vi "TPP-printer-v3.2.vi"() -> ()   [LabVIEW 2015]
uses:
  <vilib>/Math Plots/3D Math Plots/3D Scatter/3D Scatter XCtrl/3D Scatter.xctl
  <vilib>/DAQmx/write.llb/DAQmx Write (Digital Bool 1Line 1Point).vi
  <vilib>/Utility/file.llb/Read Delimited Spreadsheet (I64).vi
  <vilib>/Math Plots/3D Math Plots/3D Scatter/3D Scatter Datatype/Public/Plot Helper (Vector).vi
  <vilib>/DAQmx/create/channels.llb/DAQmx Create Channel (DO-Digital Output).vi
  <vilib>/DAQmx/miscellaneous.llb/DAQmx Fill In Error Info.vi
  <vilib>/Math Plots/3D Math Plots/3D Scatter/3D Scatter Datatype/3D Scatter Datatype.lvclass
panel:
  in  "Z轴驱动序列号":string="27002049"
  out "当前状态：":string
  in  "停止":bool
  in  "选项卡控件":enum32{"参数设置", "模型预览", "打印监控", "信息反馈"}(tab)
  in  "打印设置":T1={"f_objecitve(mm)"=1.8, "f_tubelens(mm)"=200.0, "f_scanlens(mm)"=50.0, "模型高/um"=2.0, "XY速度(um/s) "=0.0, "比例因子(V/°)"=1.0}
  in  "I/O 设置":T2={"matlab函数目录"=path "C:/Users/eason/Documents/GitHub/TPP-3D-printer/Matlab", "读取点阵文件"=path "C:/Users/eason/Documents/GitHub/TPP-3D-printer/Matlab/grating.txt", "DO通道：shutter控制"="Dev1/port1/line0", "AO通道：X前Y后"="Dev1/ao0:1", "Z轴驱动序列号"="27002049"}
  in  "刷新设置":bool
  out "三维散点图":refnum<class "3D Plot Datatype.lvclass">[](xcontrol)
  in  "取消打印":bool
  in  "开始打印":bool
  out "XYZG当前值/um":dbl[](array[numeric])=[-6.2105263157894735, -0.5263157894736842, 0.0, 1.0] format="%#.2g"
  out "每点耗时/ms":dbl=12.012958526611328 format="%#.0f"
  out "每行耗时/s":dbl=1.5567584037780762 format="%#.2g"
  out "每层耗时/min":dbl format="%#.2g"
  out "当前完成量：":u8(slide)=3 scale=0.0..100.0
  out "%":dbl=3.284878476249388 format="%#.2g"
  out "耗时/min":dbl=1.0008915185928344 format="%#.2g"
  out "三维散点图 2":refnum<class "3D Plot Datatype.lvclass">[](xcontrol)
  in  "跟踪路径":bool
  out "时刻":T3={"点时间"=timestamp(3595558893.17812 s since 1904-01-01), "行时间"=timestamp(3595558891.757594 s since 1904-01-01), "层时间"=timestamp(3595558833.124629 s since 1904-01-01)}
  out "起始时间":timestamp
  out "暂停时间/min":dbl=1.0008915185928344 format="%#.2g"
  out "当前扫描速度(um/s)":dbl
  out "XYZG坐标表":dbl[][](array[numeric])
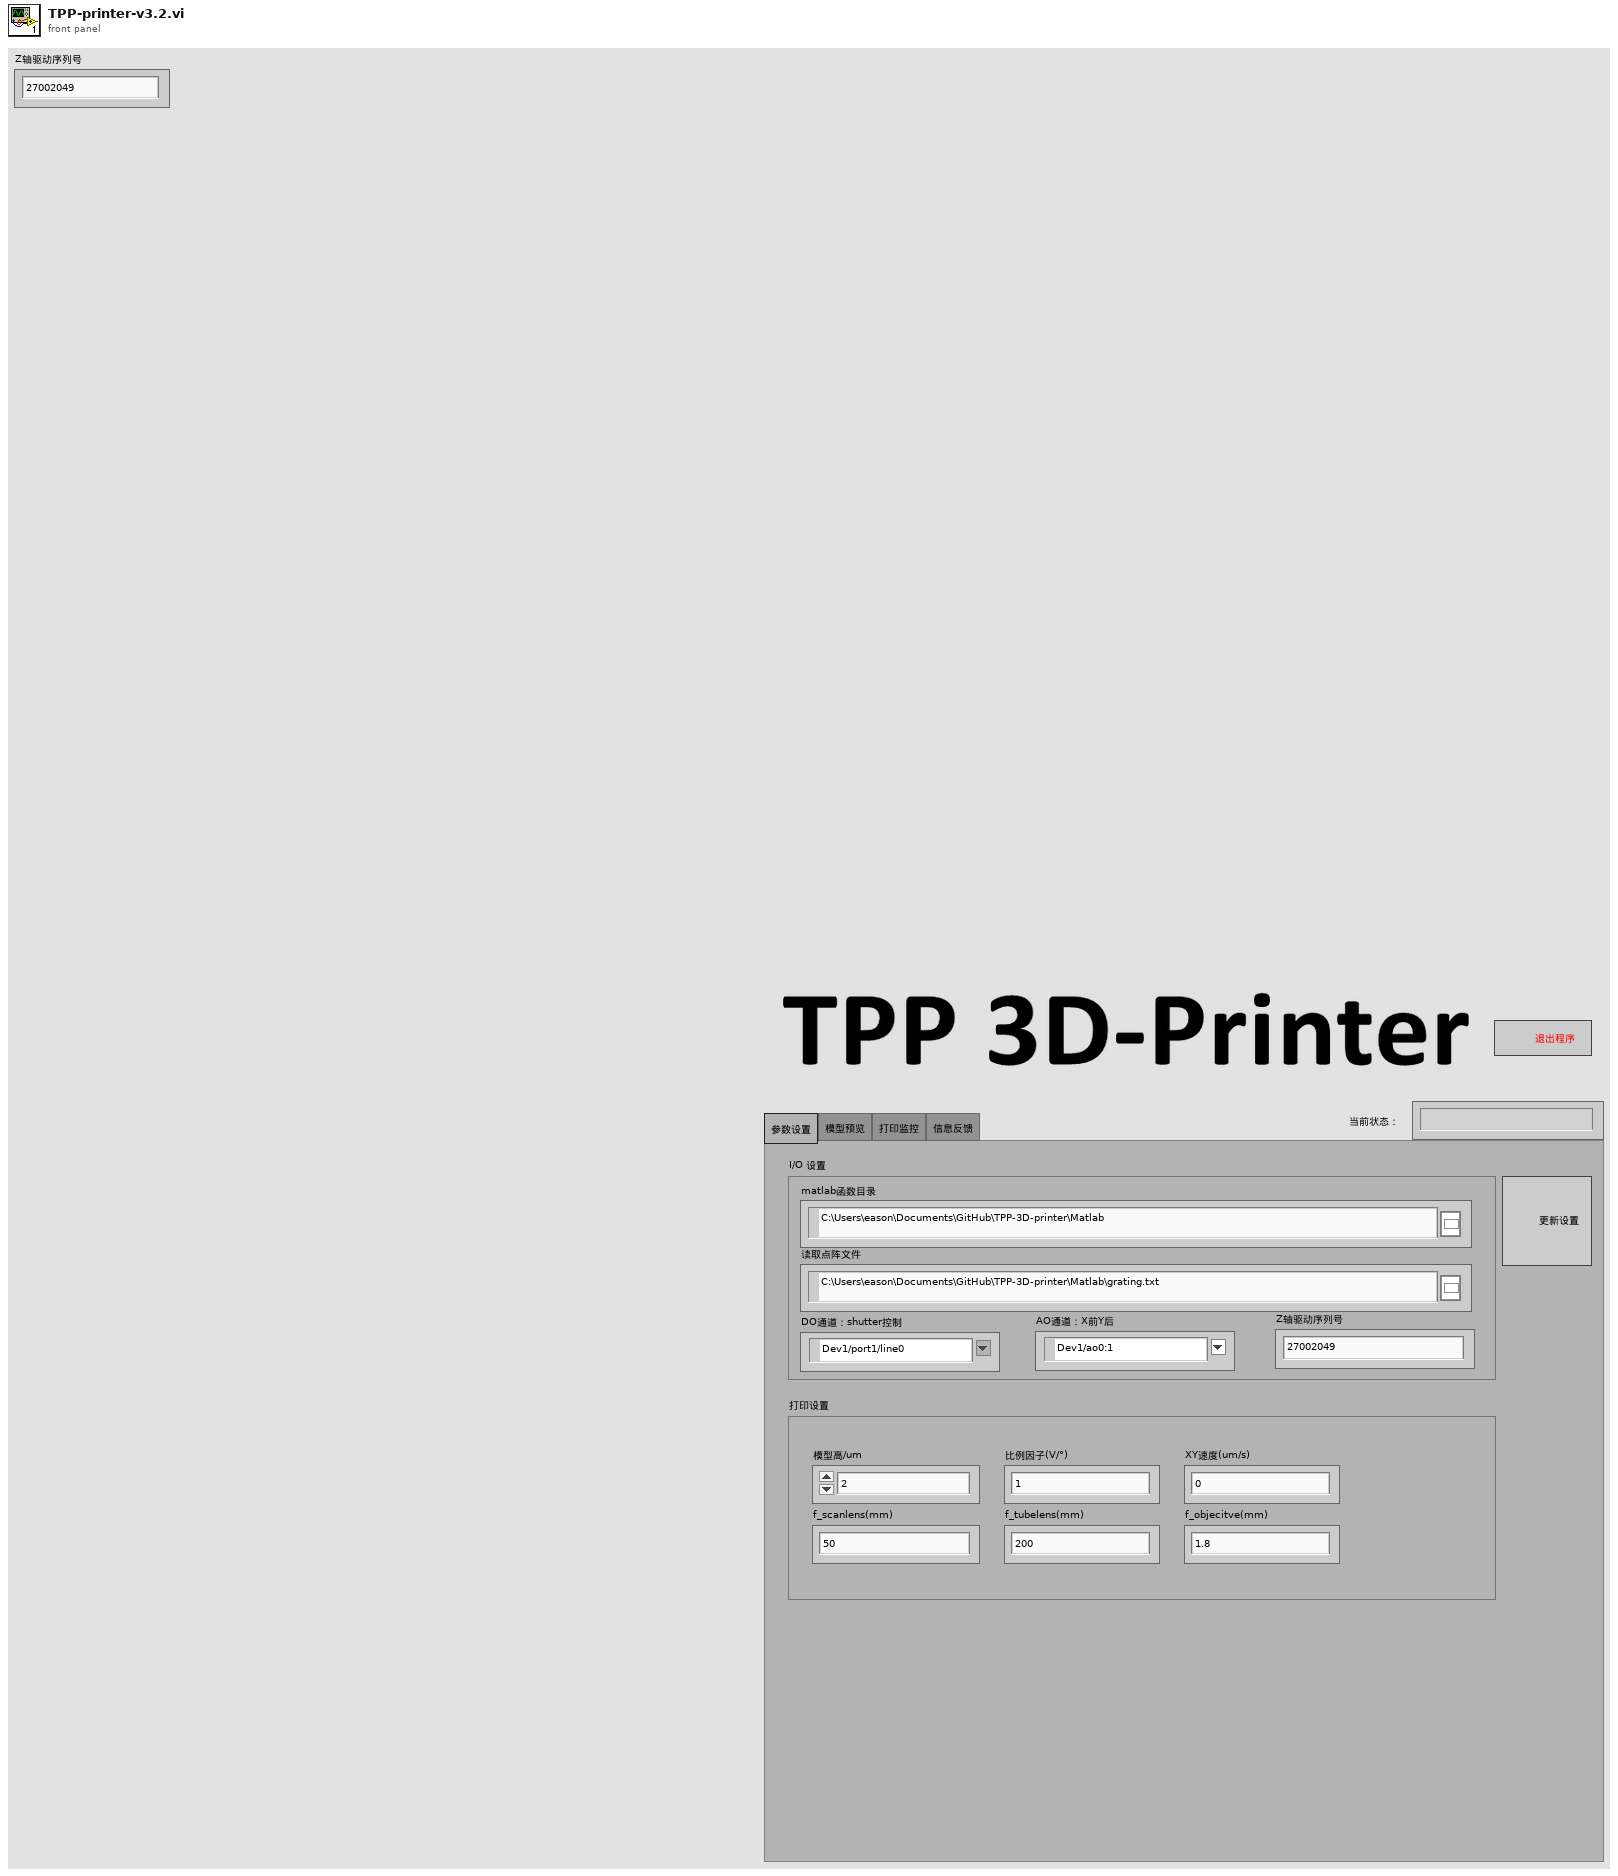
[diagram p1: front panel]
types:
  T1 = cluster{"f_objecitve(mm)":dbl, "f_tubelens(mm)":dbl, "f_scanlens(mm)":dbl, "模型高/um":dbl, "XY速度(um/s) ":dbl, "比例因子(V/°)":dbl}
  T2 = cluster{"matlab函数目录":path, "读取点阵文件":path, "DO通道：shutter控制":tag, "AO通道：X前Y后":tag, "Z轴驱动序列号":string}
  T3 = cluster{"点时间":timestamp, "行时间":timestamp, "层时间":timestamp}
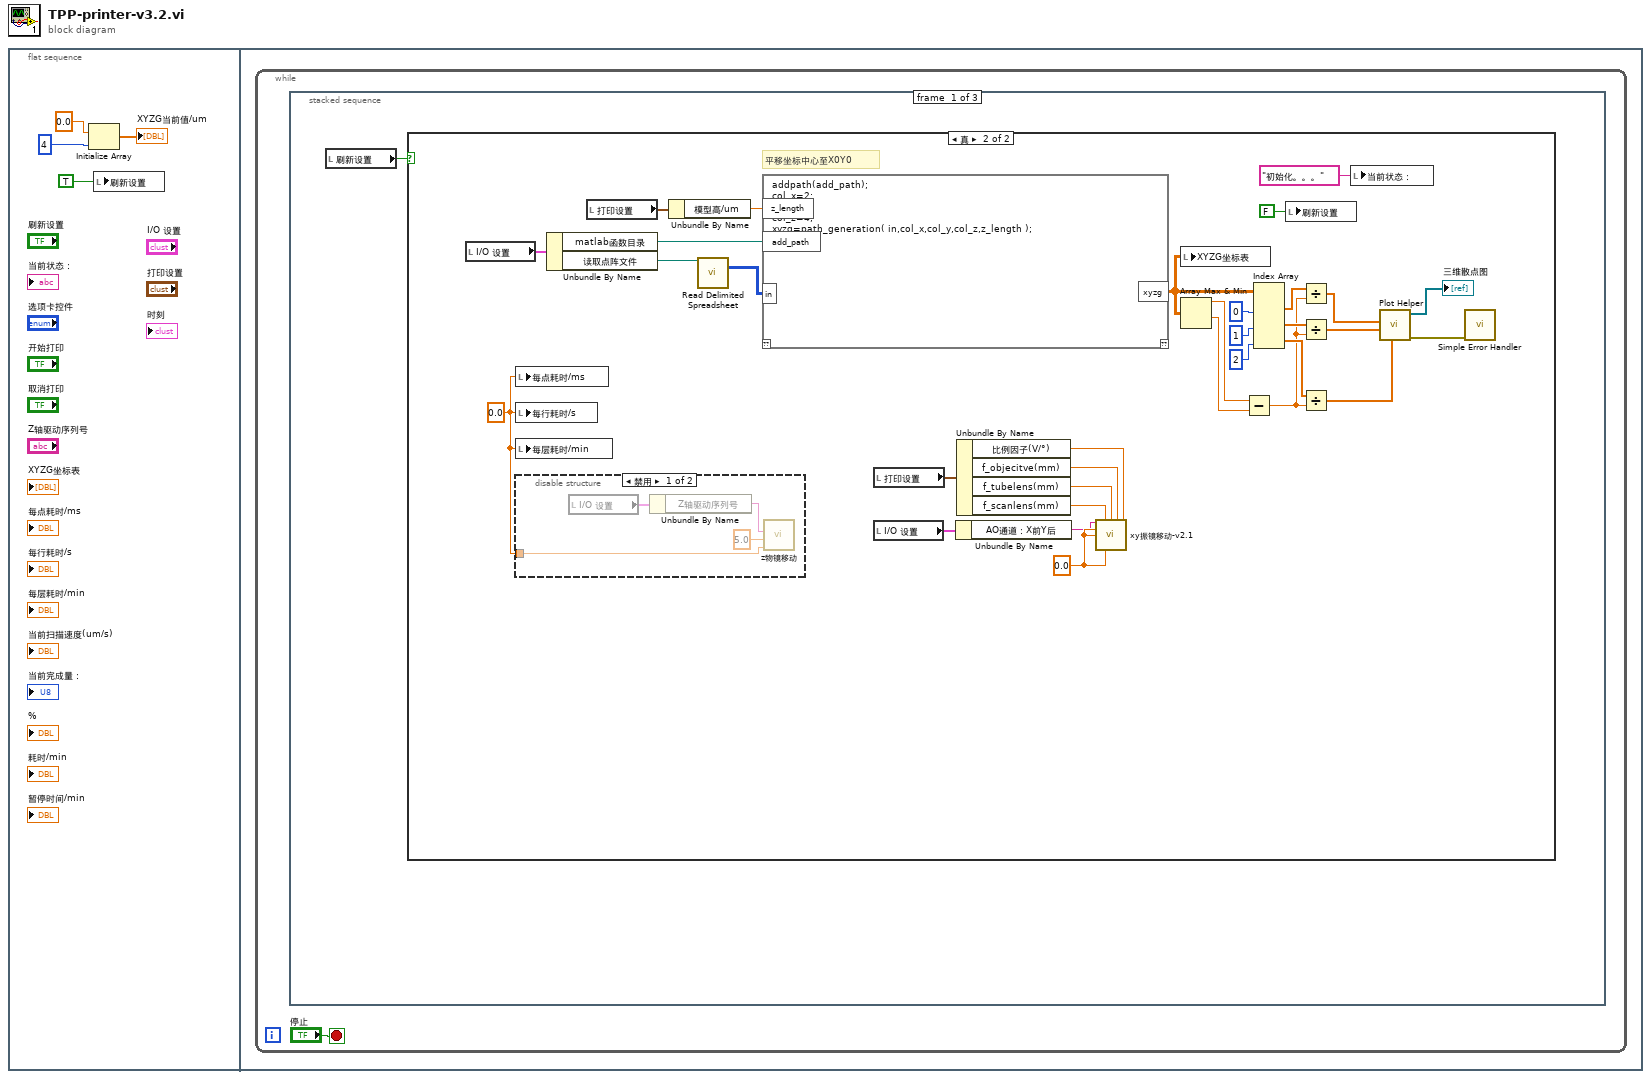
[diagram p0: block diagram]
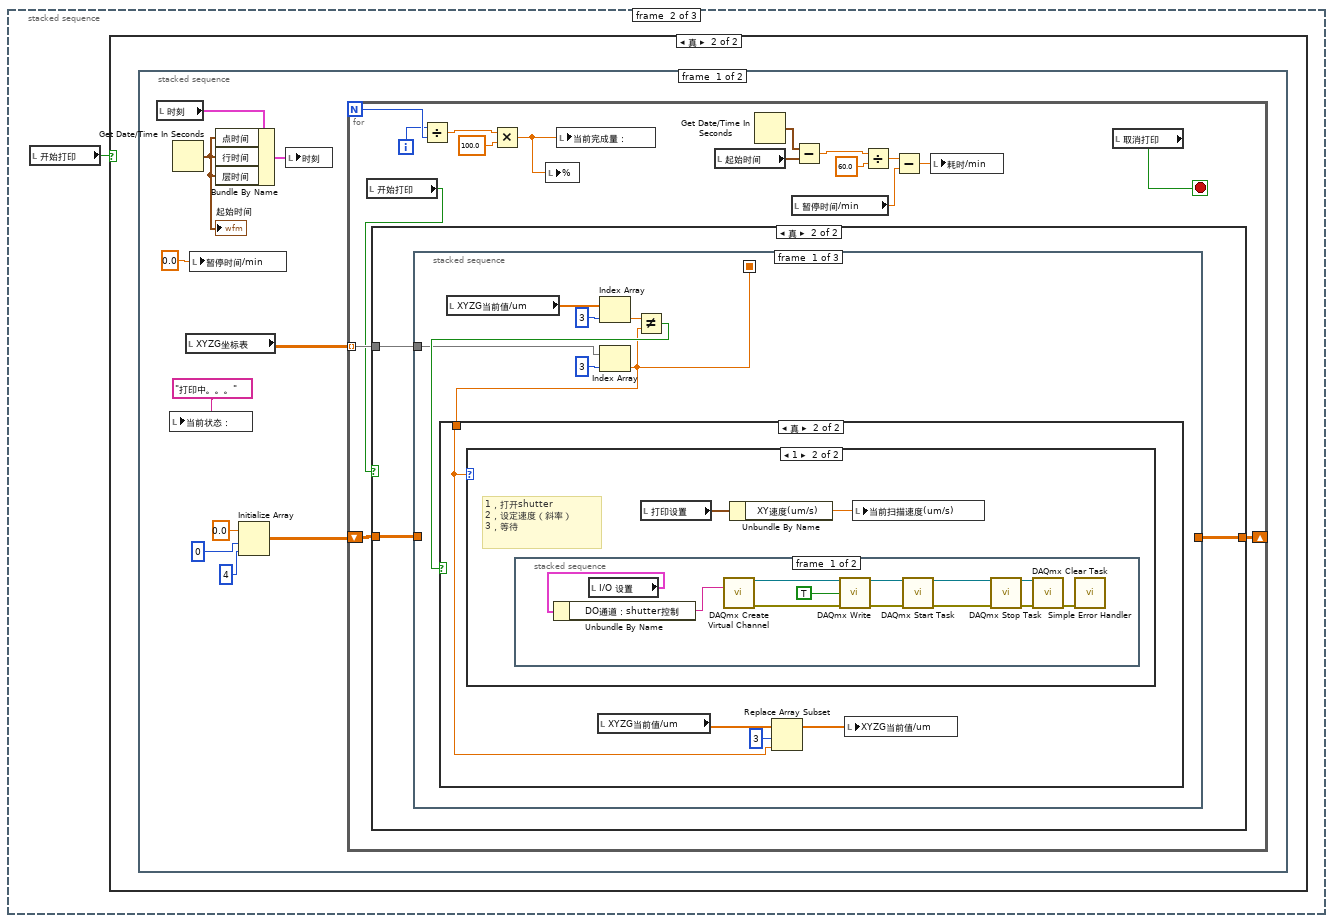
[diagram p4: hidden frame]
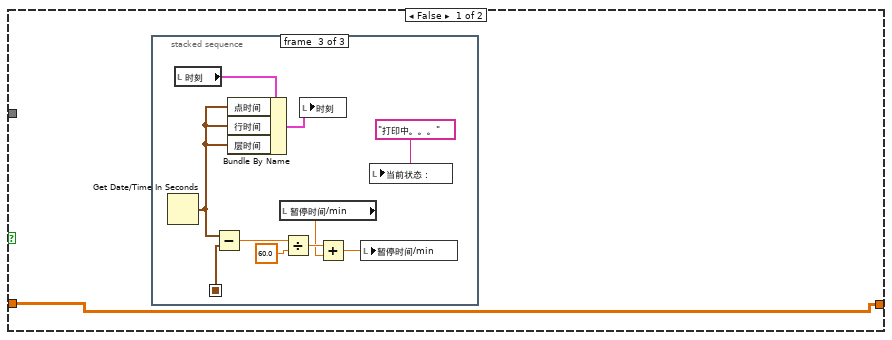
[diagram p6: hidden frame]
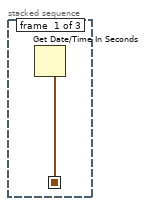
[diagram p7: hidden frame]
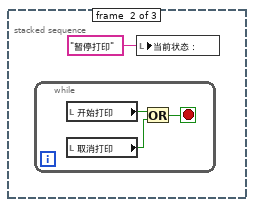
[diagram p8: hidden frame]
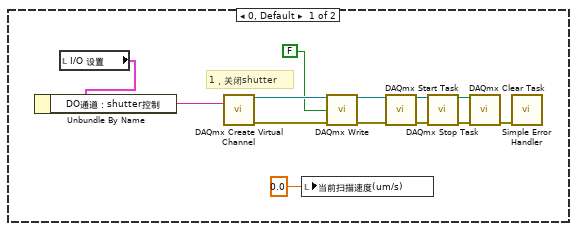
[diagram p10: hidden frame]
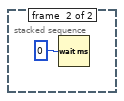
[diagram p11: hidden frame]
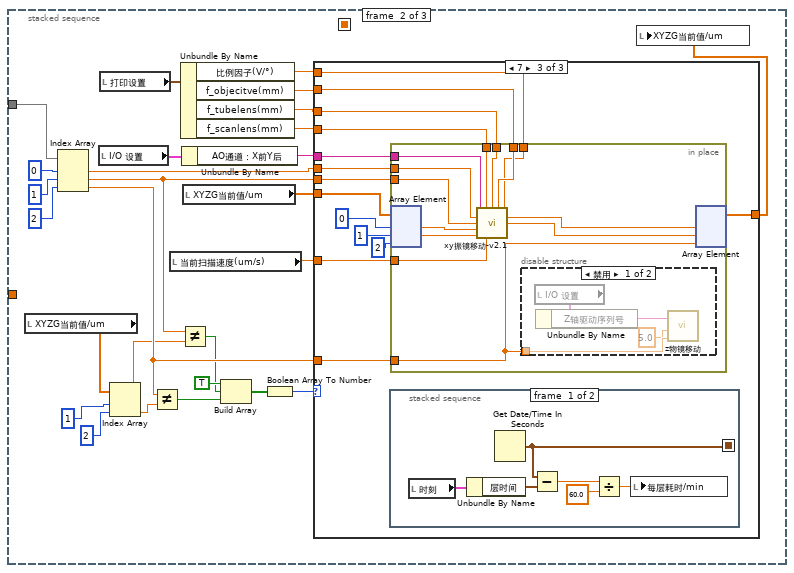
[diagram p12: hidden frame]
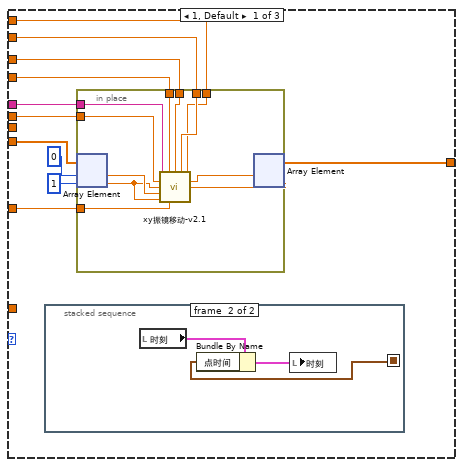
[diagram p13: hidden frame]
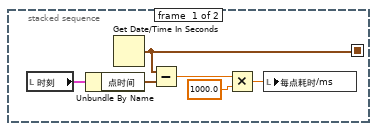
[diagram p14: hidden frame]
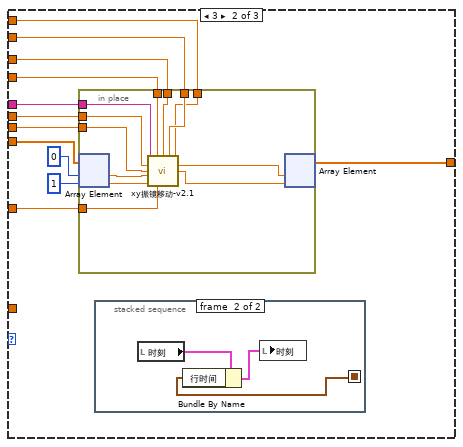
[diagram p15: hidden frame]
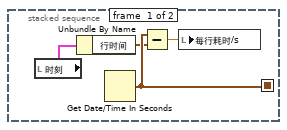
[diagram p16: hidden frame]
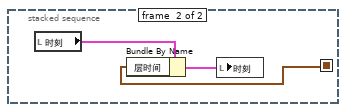
[diagram p17: hidden frame]
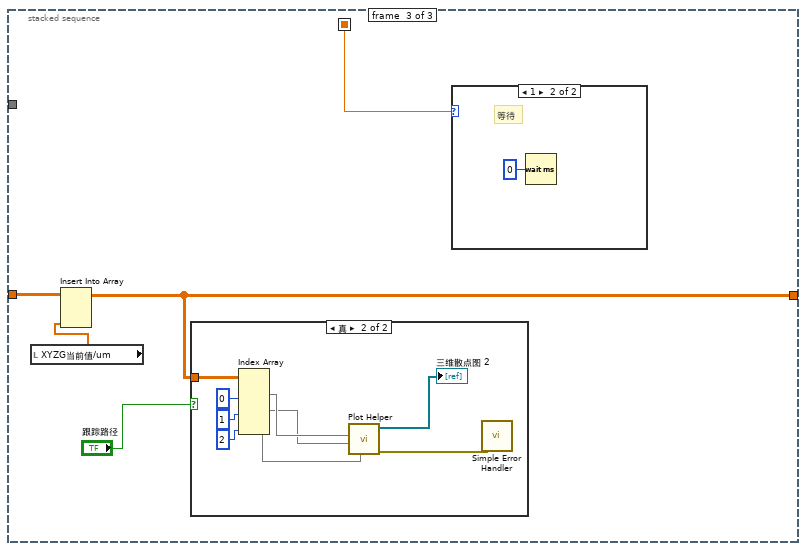
[diagram p19: hidden frame]
diagram:
  n1 = flat-sequence {
    frame #0 {
      n2 = Initialize Array(0.0 ("元素"), 4 ("维数大小")) -> (→"XYZG当前值/um":dbl[])
      n3 = local write "刷新设置"(TRUE ("刷新设置")) -> ()
    }
    frame #1 {
      n4 = while {
        stop <- "停止" stop-if-true
        n5 = stacked-sequence {
          frame #0 {
            n6 = local read "刷新设置"() -> (w6:bool)
            n7 = case shown="真" w6 {
              frame False {
              }
              frame True {
                w13 = 0.0 ("每点耗时/ms")
                w22 = 0.0 ("速度(°/s)")
                # "平移坐标中心至X0Y0"
                n8 = local read "I/O 设置"() -> (w37:T2)
                n9 = local write "每点耗时/ms"(w13) -> ()
                n10 = local write "每行耗时/s"(w13) -> ()
                n11 = local write "每层耗时/min"(w13) -> ()
                n12 = disable-structure shown="禁用" {
                  disable-tunnel: w13 -> [w42 _]
                  frame Disabled {
                    n13 = local read "I/O 设置"() -> (w40:T2)
                    n14 = Unbundle By Name(w40) -> ("Z轴驱动序列号"=w39:string)
                    n15 = call "z物镜移动.vi"("position"=w42, "maxVelocity"=5.0, "SerialNumber"=w39) -> ()  [unwired: 6 in, 3 out]
                  }
                  frame Enabled {
                  }
                }
                n16 = Unbundle By Name(w37) -> ("matlab函数目录"=w35:path, "读取点阵文件"=w36:path)
                n17 = local read "打印设置"() -> (w34:T1)
                n18 = Unbundle By Name(w34) -> ("模型高/um"=w33:dbl)
                n19 = call-poly <vilib>:"Read Delimited Spreadsheet.vi"("file path (dialog if empty)"=w36) -> ("all rows"=w38:i64[][])  [unwired: 9 in, 5 out]
                n20 = script code="addpath(add_path);\ncol_x=2;\ncol_y=3;\ncol_z=4;\nxyzg=path_generation( in,col_x,col_y,col_z,z_length );"("in"=w38, "z_length"=w33, "add_path"=w35) -> ("xyzg"=w23:dbl[][])  [unwired: 1 in, 1 out]
                n21 = local read "打印设置"() -> (w19:T1)
                n22 = local read "I/O 设置"() -> (w21:T2)
                n23 = Unbundle By Name(w21) -> ("AO通道：X前Y后"=w20:tag)
                n24 = Unbundle By Name(w19) -> ("比例因子(V/°)"=w12:dbl, "f_objecitve(mm)"=w16:dbl, "f_tubelens(mm)"=w17:dbl, "f_scanlens(mm)"=w18:dbl)
                n25 = call "xy振镜移动-v2.1.vi"("AO通道：X前Y后"=w20, "f_scanlens(mm)"=w18, "f_tubelens(mm)"=w17, "f_objecitve(mm)"=w16, "比例因子(V/°)"=w12, "x终止位(um)"=w22, "y终止位(um)"=w22, "速度(um/s)"=w22) -> ()  [unwired: 6 in, 2 out]
                n26 = local write "XYZG坐标表"(w23) -> ()
                n27 = Array Max & Min(array=w23) -> (max value=w25:dbl, min value=w26:dbl)  [unwired: 2 out]
                n28 = Subtract(x=w25, y=w26) -> (x-y=w24:dbl)
                n29 = Index Array(array=w23, index (col) #1=0 ("禁用的索引 (列)"), index (col) #2=1 ("索引 (列)"), index (col) #3=2 ("索引 (列)")) -> (element #1=w29:dbl[], element #2=w28:dbl[], element #3=w27:dbl[])  [unwired: 3 in]
                n30 = local write "刷新设置"(FALSE ("刷新设置")) -> ()
                n31 = Divide(x=w29, y=w24) -> (x/y=w8:dbl[])
                n32 = Divide(x=w28, y=w24) -> (x/y=w7:dbl[])
                n33 = Divide(x=w27, y=w24) -> (x/y=w9:dbl[])
                n34 = local write "当前状态："("初始化。。。" ("当前状态：")) -> ()
                n35 = call-poly <vilib>:"Plot Helper.vi"("z vector"=w9, "y vector"=w7, "x vector"=w8) -> ("error out"=w10:errorcluster, "3D Plot lvclass Array out"=→"三维散点图":refnum<class "3D Plot Datatype.lvclass">[])  [unwired: 3 in, 4 out]
                n36 = call <vilib>:"Simple Error Handler.vi"("error in (no error)"=w10) -> ()  [unwired: 4 in, 5 out]
              }
            }
          }
          frame #1 {
            n37 = local read "开始打印"() -> (w43:bool)
            n38 = case shown="真" w43 {
              frame False {
              }
              frame True {
                n39 = stacked-sequence {
                  frame #0 {
                    n40 = local read "时刻"() -> (w50:T3)
                    n41 = local write "当前状态："("打印中。。。" ("当前状态：")) -> ()
                    n42 = Get Date/Time In Seconds() -> (seconds since 1Jan1904=w49:timestamp)
                    "起始时间" <- w49
                    n43 = local read "XYZG坐标表"() -> (w52:dbl[][])
                    n44 = local write "暂停时间/min"(0.0 ("暂停耗时/min")) -> ()
                    n45 = Bundle By Name(cluster=w50, "点时间"=w49, "行时间"=w49, "层时间"=w49) -> (w48:T3)
                    n46 = Initialize Array(0.0 ("元素"), 0 ("维数大小"), 4 ("维数大小")) -> (w46:dbl[][])
                    n47 = local write "时刻"(w48) -> ()
                    n48 = for {
                      N -> [w69]
                      tunnel: w52 -> [w70] mode=indexing
                      shift-right: [w55] -> _
                      shift-left: w46 -> [w56]
                      i -> [w54]
                      stop <- w65 stop-if-true
                      n49 = local read "开始打印"() -> (w66:bool)
                      n50 = case shown="真" w66 {
                        tunnel: w70 -> [_ w89]
                        tunnel: w56 -> [w71 w88]
                        tunnel: [w71 w87] -> w55
                        frame False {
                          n51 = stacked-sequence {
                            seq-local: [w72 _ _] -> [_ _ w80]
                            frame #0 {
                              n52 = Get Date/Time In Seconds() -> (seconds since 1Jan1904=w72:timestamp)
                            }
                            frame #1 {
                              n53 = while {
                                stop <- w74 stop-if-true
                                n54 = local read "开始打印"() -> (w76:bool)
                                n55 = local read "取消打印"() -> (w75:bool)
                                n56 = Or(x=w76, y=w75) -> (x .or. y?=w74:bool)
                              }
                              n57 = local write "当前状态："("暂停打印" ("当前状态：")) -> ()
                            }
                            frame #2 {
                              n58 = Get Date/Time In Seconds() -> (seconds since 1Jan1904=w77:timestamp)
                              n59 = local read "时刻"() -> (w79:T3)
                              n60 = Subtract(x=w77, y=w80) -> (x-y=w85:dbl)
                              n61 = Bundle By Name(cluster=w79, "点时间"=w77, "行时间"=w77, "层时间"=w77) -> (w78:T3)
                              n62 = local read "暂停时间/min"() -> (w82:dbl)
                              n63 = Divide(x=w85, y=60.0) -> (x/y=w83:dbl)
                              n64 = local write "时刻"(w78) -> ()
                              n65 = Add(x=w83, y=w82) -> (x+y=w81:dbl)
                              n66 = local write "暂停时间/min"(w81) -> ()
                              n67 = local write "当前状态："("打印中。。。" ("当前状态：")) -> ()
                            }
                          }
                        }
                        frame True {
                          n68 = stacked-sequence {
                            seq-local: [w91 _ _] -> [_ _ w262]
                            tunnel: w89 -> [w90 w137 _]
                            tunnel: w88 -> [_ _ w261]
                            tunnel: [_ _ w258] -> w87
                            frame #0 {
                              n69 = local read "XYZG当前值/um"() -> (w94:dbl[])
                              n70 = Index Array(array=w94, index=3 ("索引")) -> (element=w92:dbl)
                              n71 = Index Array(array=w90, index=3 ("禁用的索引 (列)")) -> (element=w91:dbl)
                              n72 = Not Equal?(x=w92, y=w91) -> (x != y?=w95:bool)
                              n73 = case shown="真" w95 {
                                tunnel: w91 -> [_ w98]
                                frame False {
                                }
                                frame True {
                                n74 = case shown="1" w98 {
                                frame 0, Default {
                                # "1，关闭shutter"
                                n75 = local read "I/O 设置"() -> (w102:T2)
                                n76 = Unbundle By Name(w102) -> ("DO通道：shutter控制"=w101:tag)
                                n77 = call-poly <vilib>:"DAQmx Create Virtual Channel.vi"("lines"=w101) -> ("task out"=w113:refnum<k21>, "error out"=w112:errorcluster)  [unwired: 13 in]
                                n78 = local write "当前扫描速度(um/s)"(0.0 ("扫描速度(°/s)")) -> ()
                                n79 = call-poly <vilib>:"DAQmx Write.vi"("task/channels in"=w113, "data"=FALSE, "error in"=w112) -> ("task out"=w110:refnum<k21>, "error out"=w109:errorcluster)  [unwired: 10 in, 1 out]
                                n80 = call <vilib>:"DAQmx Start Task.vi"("task/channels in"=w110, "error in"=w109) -> ("task out"=w104:refnum<k21>, "error out"=w103:errorcluster)  [unwired: 12 in]
                                n81 = call <vilib>:"DAQmx Stop Task.vi"("task/channels in"=w104, "error in"=w103) -> ("task out"=w108:refnum<k21>, "error out"=w107:errorcluster)  [unwired: 12 in]
                                n82 = call <vilib>:"DAQmx Clear Task.vi"("task in"=w108, "error in"=w107) -> ("error out"=w106:errorcluster)  [unwired: 13 in]
                                n83 = call <vilib>:"Simple Error Handler.vi"("error in (no error)"=w106) -> ()  [unwired: 4 in, 5 out]
                                }
                                frame 1 {
                                # "1，打开shutter\n2，设定速度（斜率）\n3，等待"
                                n84 = stacked-sequence {
                                frame #0 {
                                n85 = local read "I/O 设置"() -> (w117:T2)
                                n86 = Unbundle By Name(w117) -> ("DO通道：shutter控制"=w116:tag)
                                n87 = call-poly <vilib>:"DAQmx Create Virtual Channel.vi"("lines"=w116) -> ("task out"=w127:refnum<k21>, "error out"=w126:errorcluster)  [unwired: 13 in]
                                n88 = call-poly <vilib>:"DAQmx Write.vi"("task/channels in"=w127, "data"=TRUE, "error in"=w126) -> ("task out"=w124:refnum<k21>, "error out"=w123:errorcluster)  [unwired: 10 in, 1 out]
                                n89 = call <vilib>:"DAQmx Start Task.vi"("task/channels in"=w124, "error in"=w123) -> ("task out"=w119:refnum<k21>, "error out"=w118:errorcluster)  [unwired: 12 in]
                                n90 = call <vilib>:"DAQmx Stop Task.vi"("task/channels in"=w119, "error in"=w118) -> ("task out"=w122:refnum<k21>, "error out"=w121:errorcluster)  [unwired: 12 in]
                                n91 = call <vilib>:"DAQmx Clear Task.vi"("task in"=w122, "error in"=w121) -> ("error out"=w120:errorcluster)  [unwired: 13 in]
                                n92 = call <vilib>:"Simple Error Handler.vi"("error in (no error)"=w120) -> ()  [unwired: 4 in, 5 out]
                                }
                                frame #1 {
                                n93 = Wait (ms)(milliseconds to wait=u32 0 ("等待时间（毫秒）")) -> ()  [unwired: 1 out]
                                }
                                }
                                n94 = local read "打印设置"() -> (w115:T1)
                                n95 = Unbundle By Name(w115) -> ("XY速度(um/s)"=w114:dbl)
                                n96 = local write "当前扫描速度(um/s)"(w114) -> ()
                                }
                                }
                                n97 = local read "XYZG当前值/um"() -> (w100:dbl[])
                                n98 = Replace Array Subset(array=w100, new element=w98, index=3 ("索引")) -> (w97:dbl[])
                                n99 = local write "XYZG当前值/um"(w97) -> ()
                                }
                              }
                            }
                            frame #1 {
                              n100 = local read "XYZG当前值/um"() -> (w145:dbl[])
                              n101 = Index Array(array=w137, index #1=0 ("禁用的索引 (列)"), index #2=1 ("索引"), index #3=2 ("索引")) -> (element #1=w149:dbl, element #2=w140:dbl, element #3=w144:dbl)
                              n102 = local read "I/O 设置"() -> (w131:T2)
                              n103 = local read "打印设置"() -> (w136:T1)
                              n104 = Index Array(array=w145, index #1=1 ("索引"), index #2=2 ("索引")) -> (element #1=w139:dbl, element #2=w141:dbl)
                              n105 = Not Equal?(x=w144, y=w141) -> (x != y?=w143:bool)
                              n106 = local read "当前扫描速度(um/s)"() -> (w154:dbl)
                              n107 = Not Equal?(x=w140, y=w139) -> (x != y?=w138:bool)
                              n108 = Unbundle By Name(w136) -> ("比例因子(V/°)"=w135:dbl, "f_objecitve(mm)"=w133:dbl, "f_tubelens(mm)"=w134:dbl, "f_scanlens(mm)"=w132:dbl)
                              n109 = Unbundle By Name(w131) -> ("AO通道：X前Y后"=w130:tag)
                              n110 = local read "XYZG当前值/um"() -> (w152:dbl[])
                              n111 = Build Array(TRUE ("元素"), w138, w143) -> (w151:bool[])
                              n112 = Boolean Array To Number(Boolean array=w151) -> (number=w129:u32)
                              n113 = case shown="7" w129 {
                                tunnel: w130 -> [w161 w193 w229]
                                tunnel: w149 -> [w163 w194 w228]
                                tunnel: w152 -> [w166 w195 w227]
                                tunnel: [w157 w188 w219] -> w153
                                tunnel: w154 -> [w162 w196 w226]
                                tunnel: w140 -> [_ w192 w225]
                                tunnel: w144 -> [_ _ w220]
                                tunnel: w132 -> [w160 w191 w224]
                                tunnel: w134 -> [w159 w190 w223]
                                tunnel: w133 -> [w158 w189 w222]
                                tunnel: w135 -> [w156 w187 w218]
                                frame 1, Default {
                                n114 = stacked-sequence {
                                seq-local: [w169 _] -> [_ w175]
                                frame #0 {
                                n115 = local read "时刻"() -> (w167:T3)
                                n116 = Unbundle By Name(w167) -> ("点时间"=w168:timestamp)
                                n117 = Get Date/Time In Seconds() -> (seconds since 1Jan1904=w169:timestamp)
                                n118 = Subtract(x=w169, y=w168) -> (x-y=w172:dbl)
                                n119 = Multiply(x=w172, y=1000.0) -> (x*y=w170:dbl)
                                n120 = local write "每点耗时/ms"(w170) -> ()
                                }
                                frame #1 {
                                n121 = local read "时刻"() -> (w173:T3)
                                n122 = Bundle By Name(cluster=w173, "点时间"=w175) -> (w174:T3)
                                n123 = local write "时刻"(w174) -> ()
                                }
                                }
                                n124 = in-place {
                                in-place-border: w163 -> [w181]
                                in-place-border: w162 -> [w186]
                                in-place-border: w161 -> [w185]
                                in-place-border: w160 -> [w184]
                                in-place-border: w159 -> [w183]
                                in-place-border: w158 -> [w182]
                                in-place-border: w156 -> [w176]
                                n125 = in-place-array #1(w166, 0, 1) -> (w180:dbl, w179:dbl)
                                n126 = call "xy振镜移动-v2.1.vi"("AO通道：X前Y后"=w185, "f_scanlens(mm)"=w184, "f_tubelens(mm)"=w183, "f_objecitve(mm)"=w182, "比例因子(V/°)"=w176, "x终止位(um)"=w181, "y终止位(um)"=w179, "x初始位(um)"=w180, "y初始位(um)"=w179, "速度(um/s)"=w186) -> ("x终止位(um) 2"=w178:dbl, "y终止位(um) 2"=w177:dbl)  [unwired: 4 in]
                                n127 = in-place-array #1(w178, w177) -> (w157:dbl[])  [unwired: 2 out]
                                }
                                }
                                frame 3 {
                                n128 = in-place {
                                in-place-border: w194 -> [w217]
                                in-place-border: w196 -> [w216]
                                in-place-border: w193 -> [w215]
                                in-place-border: w192 -> [w211]
                                in-place-border: w191 -> [w214]
                                in-place-border: w190 -> [w213]
                                in-place-border: w189 -> [w212]
                                in-place-border: w187 -> [w206]
                                n129 = in-place-array #2(w195, 0, 1) -> (w210:dbl, w209:dbl)
                                n130 = call "xy振镜移动-v2.1.vi"("AO通道：X前Y后"=w215, "f_scanlens(mm)"=w214, "f_tubelens(mm)"=w213, "f_objecitve(mm)"=w212, "比例因子(V/°)"=w206, "x终止位(um)"=w217, "y终止位(um)"=w211, "x初始位(um)"=w210, "y初始位(um)"=w209, "速度(um/s)"=w216) -> ("x终止位(um) 2"=w208:dbl, "y终止位(um) 2"=w207:dbl)  [unwired: 4 in]
                                n131 = in-place-array #2(w208, w207) -> (w188:dbl[])  [unwired: 2 out]
                                }
                                n132 = stacked-sequence {
                                seq-local: [w201 _] -> [_ w205]
                                frame #0 {
                                n133 = local read "时刻"() -> (w199:T3)
                                n134 = Unbundle By Name(w199) -> ("行时间"=w200:timestamp)
                                n135 = Get Date/Time In Seconds() -> (seconds since 1Jan1904=w201:timestamp)
                                n136 = Subtract(x=w201, y=w200) -> (x-y=w202:dbl)
                                n137 = local write "每行耗时/s"(w202) -> ()
                                }
                                frame #1 {
                                n138 = local read "时刻"() -> (w203:T3)
                                n139 = Bundle By Name(cluster=w203, "行时间"=w205) -> (w204:T3)
                                n140 = local write "时刻"(w204) -> ()
                                }
                                }
                                }
                                frame 7 {
                                n141 = stacked-sequence {
                                seq-local: [w237 _] -> [_ w240]
                                frame #0 {
                                n142 = local read "时刻"() -> (w232:T3)
                                n143 = Unbundle By Name(w232) -> ("层时间"=w233:timestamp)
                                n144 = Get Date/Time In Seconds() -> (seconds since 1Jan1904=w237:timestamp)
                                n145 = Subtract(x=w237, y=w233) -> (x-y=w236:dbl)
                                n146 = Divide(x=w236, y=60.0) -> (x/y=w234:dbl)
                                n147 = local write "每层耗时/min"(w234) -> ()
                                }
                                frame #1 {
                                n148 = local read "时刻"() -> (w239:T3)
                                n149 = Bundle By Name(cluster=w239, "层时间"=w240) -> (w238:T3)
                                n150 = local write "时刻"(w238) -> ()
                                }
                                }
                                n151 = in-place {
                                in-place-border: w228 -> [w252]
                                in-place-border: w226 -> [w243]
                                in-place-border: w229 -> [w253]
                                in-place-border: w225 -> [w251]
                                in-place-border: w224 -> [w246]
                                in-place-border: w223 -> [w245]
                                in-place-border: w222 -> [w244]
                                in-place-border: w220 -> [w242]
                                in-place-border: w218 -> [w241]
                                n152 = in-place-array #3(w227, 0, 1, 2) -> (w248:dbl, w247:dbl)  [unwired: 1 out]
                                n153 = call "xy振镜移动-v2.1.vi"("AO通道：X前Y后"=w253, "f_scanlens(mm)"=w246, "f_tubelens(mm)"=w245, "f_objecitve(mm)"=w244, "比例因子(V/°)"=w241, "x终止位(um)"=w252, "y终止位(um)"=w251, "x初始位(um)"=w248, "y初始位(um)"=w247, "速度(um/s)"=w243) -> ("x终止位(um) 2"=w250:dbl, "y终止位(um) 2"=w249:dbl)  [unwired: 4 in]
                                n154 = disable-structure shown="禁用" {
                                disable-tunnel: w242 -> [w257 _]
                                frame Disabled {
                                n155 = local read "I/O 设置"() -> (w255:T2)
                                n156 = Unbundle By Name(w255) -> ("Z轴驱动序列号"=w254:string)
                                n157 = call "z物镜移动.vi"("position"=w257, "maxVelocity"=5.0, "SerialNumber"=w254) -> ()  [unwired: 6 in, 3 out]
                                }
                                frame Enabled {
                                }
                                }
                                n158 = in-place-array #3(w250, w249, w242) -> (w219:dbl[])  [unwired: 3 out]
                                }
                                }
                              }
                              n159 = local write "XYZG当前值/um"(w153) -> ()
                            }
                            frame #2 {
                              n160 = local read "XYZG当前值/um"() -> (w259:dbl[])
                              n161 = Insert Into Array(array=w261, new element=w259) -> (w258:dbl[][])  [unwired: 2 in]
                              n162 = case shown="真" "跟踪路径" {
                                tunnel: w258 -> [_ w263]
                                frame False {
                                }
                                frame True {
                                n163 = Index Array(array=w263, index (col) #1=0 ("禁用的索引 (列)"), index (col) #2=1 ("索引 (列)"), index (col) #3=2 ("索引 (列)")) -> (element #1=w267:dbl[], element #2=w266:dbl[], element #3=w265:dbl[])  [unwired: 3 in]
                                n164 = call-poly <vilib>:"Plot Helper.vi"("z vector"=w265, "y vector"=w266, "x vector"=w267) -> ("error out"=w264:errorcluster, "3D Plot lvclass Array out"=→"三维散点图 2":refnum<class "3D Plot Datatype.lvclass">[])  [unwired: 3 in, 4 out]
                                n165 = call <vilib>:"Simple Error Handler.vi"("error in (no error)"=w264) -> ()  [unwired: 4 in, 5 out]
                                }
                              }
                              n166 = case shown="1" w262 {
                                frame 0, Default {
                                n167 = Wait (ms)(milliseconds to wait=u32 0 ("等待时间（毫秒）")) -> ()  [unwired: 1 out]
                                }
                                frame 1 {
                                # "等待"
                                n168 = Wait (ms)(milliseconds to wait=u32 0 ("等待时间（毫秒）")) -> ()  [unwired: 1 out]
                                }
                              }
                            }
                          }
                        }
                      }
                      n169 = Divide(x=w54, y=w69) -> (x/y=w68:dbl)
                      n170 = Multiply(x=w68, y=100.0) -> (x*y=w64:dbl)
                      n171 = local write "%"(w64) -> ()
                      n172 = local write "当前完成量："(w64) -> ()
                      n173 = local read "起始时间"() -> (w60:timestamp)
                      n174 = Get Date/Time In Seconds() -> (seconds since 1Jan1904=w61:timestamp)
                      n175 = local read "暂停时间/min"() -> (w58:dbl)
                      n176 = Subtract(x=w61, y=w60) -> (x-y=w63:dbl)
                      n177 = Divide(x=w63, y=60.0) -> (x/y=w59:dbl)
                      n178 = Subtract(x=w59, y=w58) -> (x-y=w57:dbl)
                      n179 = local write "耗时/min"(w57) -> ()
                      n180 = local read "取消打印"() -> (w65:bool)
                    }
                  }
                  frame #1 {
                    n181 = local read "I/O 设置"() -> (w275:T2)
                    n182 = Unbundle By Name(w275) -> ("DO通道：shutter控制"=w274:tag)
                    n183 = local write "开始打印"(FALSE ("取消打印")) -> ()
                    n184 = local write "取消打印"(FALSE ("开始打印")) -> ()
                    n185 = call-poly <vilib>:"DAQmx Create Virtual Channel.vi"("lines"=w274) -> ("task out"=w278:refnum<k21>, "error out"=w279:errorcluster)  [unwired: 13 in]
                    n186 = call-poly <vilib>:"DAQmx Write.vi"("task/channels in"=w278, "data"=FALSE, "error in"=w279) -> ("task out"=w281:refnum<k21>, "error out"=w282:errorcluster)  [unwired: 10 in, 1 out]
                    n187 = call <vilib>:"DAQmx Start Task.vi"("task/channels in"=w281, "error in"=w282) -> ("task out"=w286:refnum<k21>, "error out"=w287:errorcluster)  [unwired: 12 in]
                    n188 = call <vilib>:"DAQmx Stop Task.vi"("task/channels in"=w286, "error in"=w287) -> ("task out"=w283:refnum<k21>, "error out"=w284:errorcluster)  [unwired: 12 in]
                    n189 = call <vilib>:"DAQmx Clear Task.vi"("task in"=w283, "error in"=w284) -> ("error out"=w285:errorcluster)  [unwired: 13 in]
                    n190 = call <vilib>:"Simple Error Handler.vi"("error in (no error)"=w285) -> ()  [unwired: 4 in, 5 out]
                  }
                }
              }
            }
          }
          frame #2 {
            n191 = local write "当前状态："("Ready" ("当前状态：")) -> ()
          }
        }
      }
    }
  }
